vi "WaveformGraph - Colors.vi"(8 "error in":errorcluster, 10 "Ctl Refnum":refnum<vi>, 11 "Material-Scheme in":refnum<class "Material-Scheme.lvclass">) -> (0 "error out":errorcluster)   [LabVIEW 2021, in "TSC Material Theme.lvlib" / "Material-Scheme.lvclass"]
doc: "Set the colors for a waveform graph type.\n\n<b>Code Developed By:</b>\nTechnology Service Corporation\n1983 S Liberty Drive\nBloomington, IN 47403\nwww.tsc.com/atcs\n\nDeveloper:\nDaniel Coons"
uses:
  Material-Scheme.lvclass
  Material-Scheme.lvclass/Material-Scheme.ctl
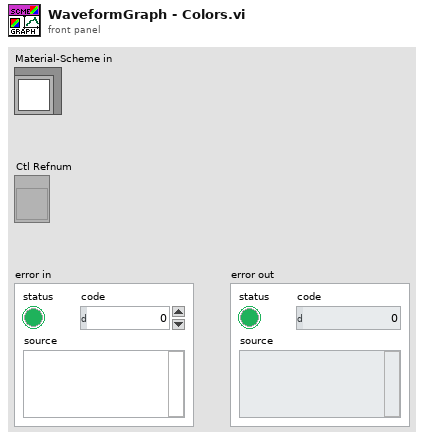
[diagram p1: front panel]
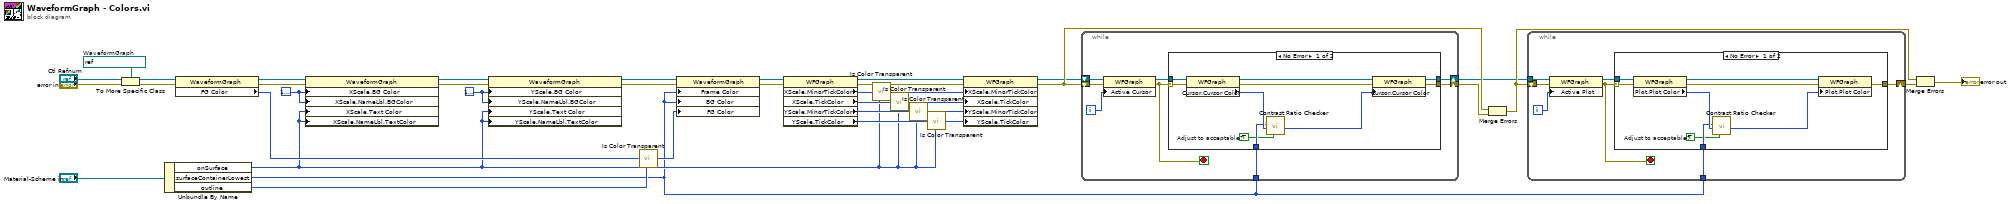
[diagram p0: block diagram]
diagram:
  w22 = u32 16777216 ("X Scale.Name Label.Colors:FG Color")
  w17 = u32 16777216 ("X Scale.Name Label.Colors:FG Color")
  w20 = refnum<vi> refnum  # WaveformGraph
  n1 = To More Specific Class(target class=w20, reference="Ctl Refnum", error in="error in") -> (specific class reference=w25:refnum<vi>, error out=w38:errorcluster)
  n2 = Unbundle By Name("Material-Scheme in") -> ("onSurface"=w6:u32, "surfaceContainerLowest"=w2:u32, "outline"=w24:u32)
  n3 = property class="WaveformGraph"(reference=w25, error in=w38) -> (reference out=w1:refnum<vi>, error out=w27:errorcluster, "FG Color"=w26:u32)
  n4 = property class="WaveformGraph"(reference=w1, error in=w27, "XScale.BG Color"=w17, "XScale.NameLbl.BGColor"=w17, "XScale.Text Color"=w6, "XScale.NameLbl.TextColor"=w6) -> (reference out=w21:refnum<vi>, error out=w36:errorcluster)
  n5 = property class="WaveformGraph"(reference=w21, error in=w36, "YScale.BG Color"=w22, "YScale.NameLbl.BGColor"=w22, "YScale.Text Color"=w6, "YScale.NameLbl.TextColor"=w6) -> (reference out=w23:refnum<vi>, error out=w37:errorcluster)
  n6 = call "Is Color Transparent.vi"("original color"=w26, "desired color"=w24) -> ("updated color"=w16:u32)  [unwired: 3 in]
  n7 = property class="WaveformGraph"(reference=w23, error in=w37, "Frame Color"=w2, "BG Color"=w2, "FG Color"=w16) -> (reference out=w15:refnum<vi>, error out=w32:errorcluster)
  n8 = property class="WFGraph"(reference=w15, error in=w32) -> (reference out=w5:refnum<vi>, error out=w31:errorcluster, "XScale.MinorTickColor"=w14:u32, "XScale.TickColor"=w12:u32, "YScale.MinorTickColor"=w10:u32, "YScale.TickColor"=w8:u32)
  n9 = call "Is Color Transparent.vi"("original color"=w14, "desired color"=w6) -> ("updated color"=w13:u32)  [unwired: 3 in]
  n10 = call "Is Color Transparent.vi"("original color"=w12, "desired color"=w6) -> ("updated color"=w11:u32)  [unwired: 3 in]
  n11 = call "Is Color Transparent.vi"("original color"=w10, "desired color"=w6) -> ("updated color"=w9:u32)  [unwired: 3 in]
  n12 = call "Is Color Transparent.vi"("original color"=w8, "desired color"=w6) -> ("updated color"=w7:u32)  [unwired: 3 in]
  n13 = property class="WFGraph"(reference=w5, error in=w31, "XScale.MinorTickColor"=w13, "XScale.TickColor"=w11, "YScale.MinorTickColor"=w9, "YScale.TickColor"=w7) -> (reference out=w4:refnum<vi>, error out=w29:errorcluster)
  n14 = while {
    shift-right: [w44] -> w28
    shift-left: w29 -> [w46]
    tunnel: w2 -> [w41]
    shift-right: [w39] -> w3
    shift-left: w4 -> [w40]
    i -> [w43]
    stop <- w45 stop-if-true
    n15 = property class="WFGraph"(reference=w40, error in=w46, "Active Cursor"=w43) -> (reference out=w42:refnum<vi>, error out=w45:errorcluster)
    n16 = case shown="No Error" w45 {
      selector: w45 -> [w56 _]
      tunnel: [w54 _] -> w44
      tunnel: w42 -> [w53 w57]
      tunnel: w41 -> [w51 _]
      tunnel: [w47 w57] -> w39
      frame No Error {
        w50 = TRUE  # Adjust to acceptable?
        n17 = property class="WFGraph"(reference=w53, error in=w56) -> (reference out=w49:refnum<vi>, error out=w55:errorcluster, "Cursor.Cursor Color"=w52:u32)
        n18 = call "Contrast Ratio Checker.vi"("Adjust to acceptable?"=w50, "On Color"=w52, "Background Color"=w51) -> ("Adjusted Color"=w48:u32)  [unwired: 6 in, 2 out]
        n19 = property class="WFGraph"(reference=w49, error in=w55, "Cursor.Cursor Color"=w48) -> (reference out=w47:refnum<vi>, error out=w54:errorcluster)
      }
      frame Error {
      }
    }
  }
  n20 = Merge Errors(w29, w28) -> (w30:errorcluster)
  n21 = while {
    shift-right: [w62] -> w34
    shift-left: w30 -> [w64]
    tunnel: w2 -> [w59]
    tunnel: w3 -> [w58]
    i -> [w61]
    stop <- w63 stop-if-true
    n22 = property class="WFGraph"(reference=w58, error in=w64, "Active Plot"=w61) -> (reference out=w60:refnum<vi>, error out=w63:errorcluster)
    n23 = case shown="No Error" w63 {
      selector: w63 -> [w73 _]
      tunnel: [w71 _] -> w62
      tunnel: w60 -> [w70 _]
      tunnel: w59 -> [w68 _]
      frame No Error {
        w67 = TRUE  # Adjust to acceptable?
        n24 = property class="WFGraph"(reference=w70, error in=w73) -> (reference out=w66:refnum<vi>, error out=w72:errorcluster, "Plot.Plot Color"=w69:u32)
        n25 = call "Contrast Ratio Checker.vi"("Adjust to acceptable?"=w67, "On Color"=w69, "Background Color"=w68) -> ("Adjusted Color"=w65:u32)  [unwired: 6 in, 2 out]
        n26 = property class="WFGraph"(reference=w66, error in=w72, "Plot.Plot Color"=w65) -> (error out=w71:errorcluster)  [unwired: 1 out]
      }
      frame Error {
      }
    }
  }
  n27 = Merge Errors(w30, w34) -> (→"error out":errorcluster)
